vi "Initialize.vi"(8 "error in (no error)":errorcluster, 11 "Serial in":refnum<class "ICPCON M-7024.lvclass">) -> (0 "error out":errorcluster, 3 "MB_TCP out":refnum<class "ICPCON M-7024.lvclass">)   [LabVIEW 2021, in "ICPCON M-7024.lvclass"]
uses:
  ICPCON M-7024.lvclass
  D:/my_projects/projects/Algorithms/Labview/21/Master CR/Master CR.lvclass
  Param/TCP Param/TCP Param.lvclass
  Modbus_v121c/Network Protocol/Network Master/Serial/Serial Master.lvclass
  D:/my_projects/projects/Algorithms/Labview/21/Modbus_v121c/Network Protocol/Network Master/Network Master.lvclass
  D:/my_projects/projects/Algorithms/Labview/21/Modbus_v121c/Network Protocol/Network Protocol.lvclass
  Modbus_v121c/Transmission Data Unit/RTU/RTU Data Unit.lvclass
  D:/my_projects/projects/Algorithms/Labview/21/Modbus_v121c/Transmission Data Unit/Serial Interface/Serial Data Unit.lvclass
  Modbus_v121c/Transmission Data Unit/Transmission Data Unit.lvclass/Transmission Data Unit.ctl
  Master CR.lvclass/Master CR.ctl
  Param/TCP Param/TCP Param.lvclass/TCP Param.ctl
  Modbus_v121c/Transmission Data Unit/Serial Interface/Serial Data Unit.lvclass/Serial Data Unit.ctl
  Modbus_v121c/Network Protocol/Network Master/Network Master.lvclass/Network Master.ctl
  Modbus_v121c/Transmission Data Unit/Serial Interface/Write timeout.vi
  Modbus_v121c/Transmission Data Unit/Serial Interface/Write baud rate.vi
  Modbus_v121c/Transmission Data Unit/Serial Interface/Write flow control.vi
  Modbus_v121c/Transmission Data Unit/Serial Interface/Write parity.vi
  Modbus_v121c/Transmission Data Unit/Serial Interface/Write visa resource name.vi
  Modbus_v121c/Transmission Data Unit/Serial Interface/Serial Data Unit.lvclass
  D:/my_projects/projects/Algorithms/Labview/21/Modbus_v121c/Transmission Data Unit/Transmission Data Unit.lvclass
  Modbus_v121c/Transmission Data Unit/ASCII/ASCII Data Unit.lvclass
  ICPCON M-7024.lvclass/ICPCON M-7024.ctl
  Serial/Serial.lvclass
  Modbus_v121c/Transmission Data Unit/Transmission Data Unit.lvclass
  Modbus_v121c/Network Protocol/Network Master/Network Master.lvclass
  Master CR.lvclass
  D:/my_projects/projects/Algorithms/Labview/21/Master CR/Devices/Serial/Serial.lvclass
  D:/my_projects/projects/Algorithms/Labview/21/Master CR/Devices/M7000/ICPCON M-7024/ICPCON M-7024.lvclass
  Modbus_v121c/Master Function Definition/Master Function Definition.lvclass
  D:/my_projects/projects/Algorithms/Labview/21/Modbus_v121c/Transmission Data Unit/RTU/RTU Data Unit.lvclass
  D:/my_projects/projects/Algorithms/Labview/21/Modbus_v121c/Transmission Data Unit/ASCII/ASCII Data Unit.lvclass
  D:/my_projects/projects/Algorithms/Labview/21/Modbus_v121c/Network Protocol/Network Master/Serial/Serial Master.lvclass
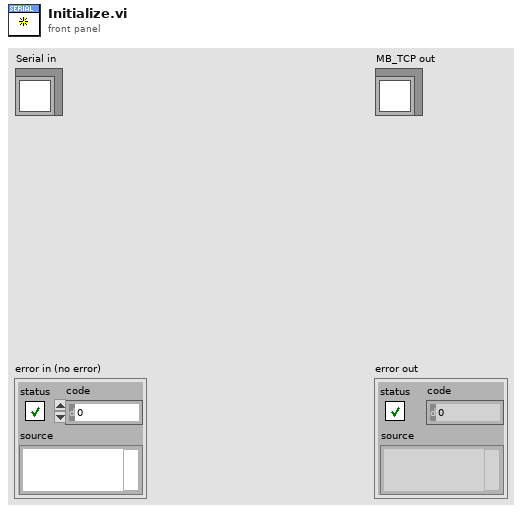
[diagram p1: front panel]
types:
  T1 = typedef "Param.lvlib/TCP Param.lvclass/timeouts.ctl" = cluster{"conn_timeout":i32, "reconn_timeout":i32, "N attempt max":i32, "t_reset_TTL":i32, "write_timeout":i32, "read_timeout":i32, "period":i32}
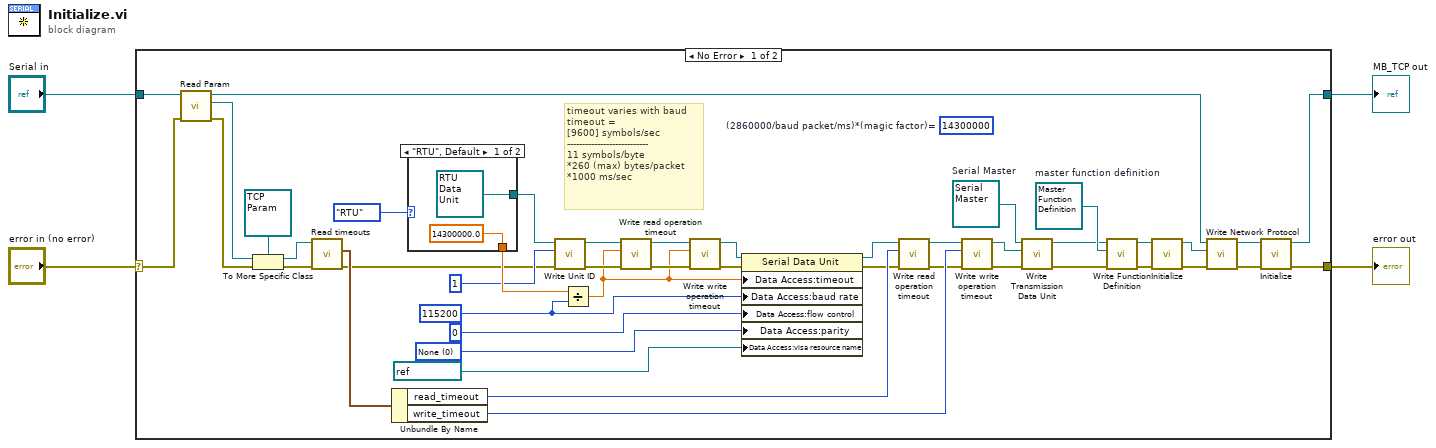
[diagram p0: block diagram]
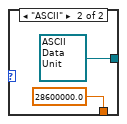
[diagram p2: hidden frame]
diagram:
  n1 = case shown="No Error" "error in (no error)" {
    selector: "error in (no error)" -> [w47 w54]
    tunnel: [w41 w54] -> w1
    tunnel: [w42 w55] -> w2
    tunnel: "Serial in" -> [w16 w55]
    frame No Error {
      w9 = refnum<class "Master Function Definition.lvclass"> refnum  # master function definition
      w15 = refnum<class "Serial Master.lvclass"> refnum  # Serial Master
      w27 = u16 0 items=["None", "Odd", "Even"] ("parity (Even)")
      w21 = u32 115200 ("baud rate (9600)")
      (unwired) u32 14300000  # (2860000/baud packet/ms)*(magic factor)=
      # "timeout varies with baud\ntimeout =\n[9600] symbols/sec\n---------------------------\n11 symbols/byte\n*260 (max) bytes/packet\n*1000 ms/sec"
      n2 = call "Read Param.vi"("error in (no error)"=w47, "MB_TCP in"=w16) -> ("error out"=w46:errorcluster, "Param"=w44:refnum<class "Param.lvclass">, "MB_TCP out"=w14:refnum<class "ICPCON M-7024.lvclass">)  [unwired: 7 in]
      n3 = To More Specific Class(target class=refnum<class "TCP Param.lvclass"> refnum ("Param.lvlib:TCP Param.lvclass"), reference=w44, error in=w46) -> (specific class reference=w45:refnum<class "TCP Param.lvclass">, error out=w48:errorcluster)
      n4 = call "Read timeouts.vi"("error in (no error)"=w48, "MBParam in"=w45) -> ("error out"=w17:errorcluster, "timeouts"=w43:T1)  [unwired: 7 in, 1 out]
      n5 = Unbundle By Name(w43) -> ("read_timeout"=w40:i32, "write_timeout"=w39:i32)
      n6 = case shown="\"RTU\", Default" enum16{"RTU", "ASCII"}."RTU" ("serial type") {
        tunnel: [refnum<class "RTU Data Unit.lvclass"> refnum ("RTU Data Unit") refnum<class "ASCII Data Unit.lvclass"> refnum ("ASCII Data Unit")] -> w36
        tunnel: [14300000.0 ("x") 28600000.0 ("x")] -> w31
        frame "RTU", Default {
        }
        frame "ASCII" {
        }
      }
      n7 = call "Write Unit ID.vi"("error in"=w17, "unit ID"=u8 1, "transmission data unit in"=w36) -> ("error out"=w32:errorcluster, "transmission data unit out"=w35:refnum<class "Serial Data Unit.lvclass">)  [unwired: 7 in]
      n8 = Divide(x=w31, y=w21) -> (x/y=w30:dbl)
      n9 = call "Write read operation timeout.vi"("error in (no error)"=w32, "read operation timeout"=w30, "transmission data unit in"=w35) -> ("error out"=w33:errorcluster, "transmission data unit out"=w34:refnum<class "Serial Data Unit.lvclass">)  [unwired: 7 in]
      n10 = call "Write write operation timeout.vi"("error in (no error)"=w33, "write operation timeout"=w30, "transmission data unit in"=w34) -> ("error out"=w22:errorcluster, "transmission data unit out"=w20:refnum<class "Serial Data Unit.lvclass">)  [unwired: 7 in]
      n11 = property class="Serial Data Unit"(reference=w20, error in=w22, "Data Access:timeout"=w30, "Data Access:baud rate"=w21, "Data Access:flow control"=u16 0 ("Flow Control"), "Data Access:parity"=w27, "Data Access:visa resource name"=refnum<visa-resource-name> "COM18" ("VISA resource name")) -> (reference out=w18:refnum<class "Serial Data Unit.lvclass">, error out=w19:errorcluster)
      n12 = call "Write read operation timeout.vi"("error in (no error)"=w19, "read operation timeout"=w40, "transmission data unit in"=w18) -> ("error out"=w37:errorcluster, "transmission data unit out"=w38:refnum<class "Serial Data Unit.lvclass">)  [unwired: 7 in]
      n13 = call "Write write operation timeout.vi"("error in (no error)"=w37, "write operation timeout"=w39, "transmission data unit in"=w38) -> ("error out"=w23:errorcluster, "transmission data unit out"=w24:refnum<class "Serial Data Unit.lvclass">)  [unwired: 7 in]
      n14 = call "Write Transmission Data Unit.vi"("error in (no error)"=w23, "Transmission Data Unit"=w24, "Network Master in"=w15) -> ("error out"=w6:errorcluster, "Network Master out"=w5:refnum<class "Serial Master.lvclass">)  [unwired: 7 in]
      n15 = call "Write Function Definition.vi"("error in"=w6, "master function definition"=w9, "Modbus master in"=w5) -> ("error out"=w8:errorcluster, "Modbus master in"=w7:refnum<class "Serial Master.lvclass">)  [unwired: 7 in]
      n16 = call-dynamic "Initialize.vi"("error in"=w8, "Serial Master in"=w7) -> ("error out"=w11:errorcluster, "Serial Master out"=w10:refnum<class "Serial Master.lvclass">)  [unwired: 8 in]
      n17 = call "Write Network Protocol.vi"("error in (no error)"=w11, "Network Protocol"=w10, "Master CR in"=w14) -> ("error out"=w13:errorcluster, "Master CR in"=w12:refnum<class "ICPCON M-7024.lvclass">)  [unwired: 7 in]
      n18 = call-parent "Initialize.vi"("error in (no error)"=w13, "Serial in"=w12) -> ("error out"=w41:errorcluster, "MB_TCP out"=w42:refnum<class "ICPCON M-7024.lvclass">)  [unwired: 8 in]
    }
    frame Error {
    }
  }
  "error out" <- w1
  "MB_TCP out" <- w2
